vi "Read FC2 Force Sensor.vi"(8 "error in (no error)":errorcluster, 11 "Model in":refnum<class "Model.lvclass">) -> (0 "error out":errorcluster, 3 "Model out":refnum<class "Model.lvclass">)   [LabVIEW 2015, in "Model.lvclass"]
uses:
  Model.lvclass
  ILC ADC/ILC ADC Factory/ILC ADC Factory.lvclass
  Model.lvclass/Model.ctl
  ILC ADC/ILC ADC/ILC ADC.lvclass
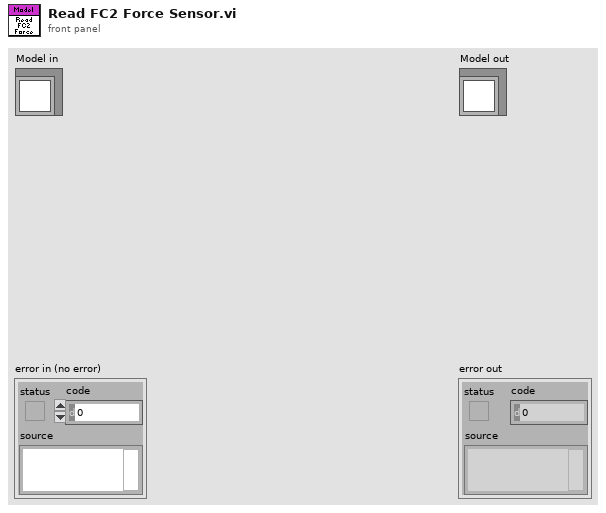
[diagram p1: front panel]
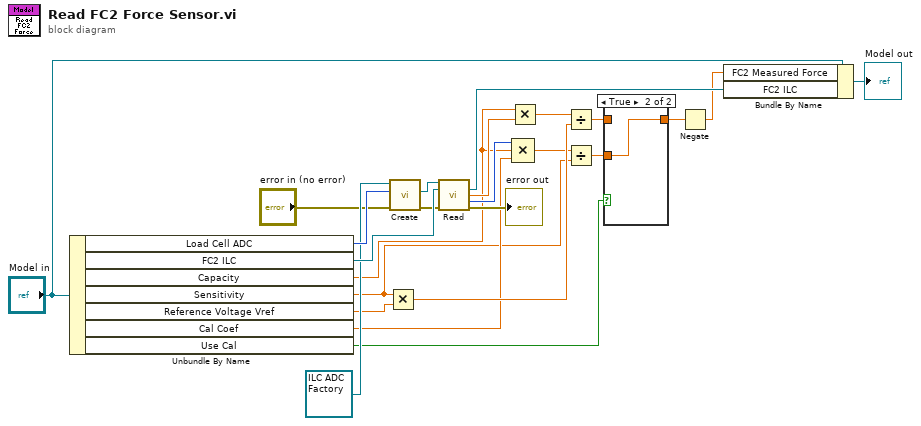
[diagram p0: block diagram]
diagram:
  n1 = Unbundle By Name("Model in") -> ("Load Cell ADC"=w24:u8, "FC2 ILC"=w22:refnum<class "ILC.lvclass">, "Capacity"=w8:dbl[unit], "Sensitivity"=w6:dbl[unit], "Reference Voltage Vref"=w11:dbl[unit], "Cal Coef"=w7:dbl, "Use Cal"=w3:bool)
  n2 = Multiply(x=w6, y=w11) -> (x*y=w13:dbl[unit])
  n3 = call-dynamic "Create.vi"("error in (no error)"="error in (no error)", "Channel"=w24, "ILC ADC Factory in"=refnum<class "ILC ADC Factory.lvclass"> refnum ("ILCADCFactory in")) -> ("error out"=w18:errorcluster, "ILC ADC"=w23:refnum<class "ILC ADC.lvclass">)  [unwired: 6 in, 1 out]
  n4 = call-dynamic "Read.vi"("ILC ADC in"=w23, "ILC In"=w22, "error in (no error)"=w18) -> ("ILC Out"=w21:refnum<class "ILC.lvclass">, "Value"=w12:dbl[unit], "N"=w9:i32, "error out"=→"error out":errorcluster)  [unwired: 8 in, 1 out]
  n5 = Multiply(x=w8, y=w12) -> (x*y=w14:dbl[unit])
  n6 = Compound Arithmetic op=MULTIPLY(w9, w8, w7) -> (w5:dbl[unit])
  n7 = Divide(x=w14, y=w13) -> (x/y=w2:dbl[unit])
  n8 = Divide(x=w5, y=w6) -> (x/y=w4:dbl[unit])
  n9 = case shown="True" w3 {
    tunnel: w4 -> [_ w26]
    tunnel: w2 -> [w25 _]
    tunnel: [w25 w26] -> w1
    frame False {
    }
    frame True {
    }
  }
  n10 = Negate(x=w1) -> (-x=w10:dbl[unit])
  n11 = Bundle By Name(cluster="Model in", "FC2 Measured Force"=w10, "FC2 ILC"=w21) -> (→"Model out":refnum<class "Model.lvclass">)
